vi "GetExeName.vi"(11 "Path":path) -> (3 "new path":path)   [LabVIEW 2017]
uses:
  Mic/Mic_Global.vi
panel:
  out "error out":errorcluster
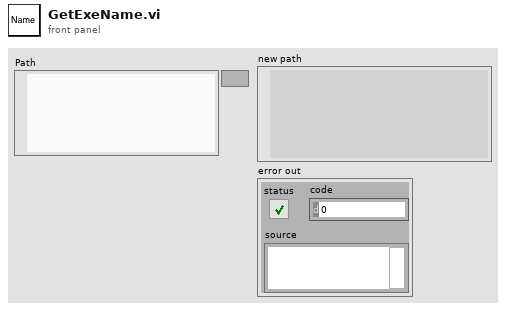
[diagram p1: front panel]
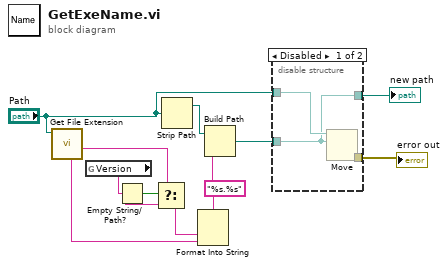
[diagram p0: block diagram]
diagram:
  n1 = call <vilib>:"Get File Extension.vi"("file"="Path") -> ("filename without extension"=w6:string, "unmodified file extension"=w9:string)  [unwired: 6 in, 3 out]
  n2 = global read "Mic_Global.vi" "Version"() -> (w4:string)
  n3 = Empty String/Path?(string/path=w4) -> (empty?=w7:bool)
  n4 = Select(t=w6, s=w7, f=w4) -> (s? t:f=w5:string)
  n5 = Strip Path(path="Path") -> (stripped path=w11:path)  [unwired: 1 out]
  n6 = Format Into String(format string="%s.%s", w5, w9) -> (resulting string=w8:string)  [unwired: 2 in, 1 out]
  n7 = Build Path(base path=w11, name or relative path=w8) -> (appended path=w3:path)
  n8 = disable-structure shown="Disabled" {
    disable-tunnel: "Path" -> [w15 w16]
    disable-tunnel: w3 -> [w13 _]
    disable-tunnel: [w14 _] -> w2
    disable-tunnel: [w13 w16] -> w1
    frame Disabled {
      n9 = Move(source path=w15, 10:w13) -> (error out=w14:errorcluster)  [unwired: 3 in, 2 out]
    }
    frame Enabled {
    }
  }
  "new path" <- w1
  "error out" <- w2
